vi "3.1.vi"() -> ()   [LabVIEW 2017]
panel:
  out "cos(x)":dbl
  out "sin(x)":dbl
  in  "x":dbl
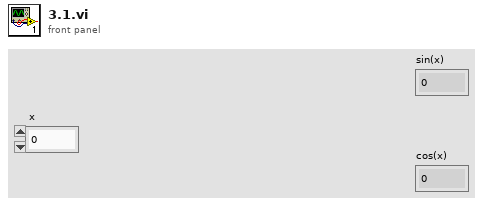
[diagram p1: front panel]
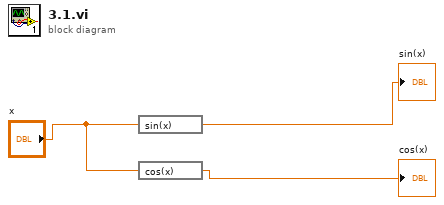
[diagram p0: block diagram]
diagram:
  n1 = expression code="sin(x)"("x") -> (→"sin(x)":dbl)
  n2 = expression code="cos(x)"("x") -> (→"cos(x)":dbl)
